vi "Practica1.vi"() -> ()   [LabVIEW 2021]
uses:
  <vilib>/imath/engines/lvmath2/RunTimeEngine/Managers/WorkSpace/UID Generator.vi
  <vilib>/imath/engines/lvmath2/RunTimeEngine/RunTimeType/NIMS_RunTimeType_From StrictType (excl LVString).vi
  <instcachedir>/0/NIMS_RunTimeType_From StrictType (excl LVString)_F2DF8362C4A748C4A5A87B97B2A722F9.lvgen/NIMS_RunTimeType_From StrictType (excl LVString)_F2DF8362C4A748C4A5A87B97B2A722F9_000.vi
  <vilib>/imath/engines/lvmath2/RunTimeEngine/LocalVariableDefStatement/MC_LocalVariableDefStatement_Display.vi
  <vilib>/imath/engines/lvmath2/RunTimeEngine/Managers/SymbolTable/Clear UID.vi
  <vilib>/imath/engines/lvmath2/RunTimeEngine/NodeEndStatement/NIMS_NodeEndStatement_Output.vi
  <instcachedir>/0/NIMS_NodeEndStatement_Output_53EC0D466D134D7ABD903AC30B43404B.lvgen/NIMS_NodeEndStatement_Output_53EC0D466D134D7ABD903AC30B43404B_001.vi
  <vilib>/imath/engines/lvmath2/RunTimeEngine/ErrorHandling/NIMS_Finalize Error.vi
  <vilib>/imath/engines/lvmath2/RunTimeEngine/ArithmeticOperatorToken/NIMS_ArithmeticOperator_power(S).vi
  <instcachedir>/0/NIMS_ArithmeticOperator_power(S)_149E20C93FA648E196B974450BC90546.lvgen/NIMS_ArithmeticOperator_power(S)_149E20C93FA648E196B974450BC90546_010.vi
  <vilib>/imathl/engines/lvmath/Functions/Error Handling/Create Error.vi
  <vilib>/imath/engines/lvmath2/RunTimeEngine/BuiltInFunctions/sin/NIMS_sin(C).vi
  <instcachedir>/0/NIMS_sin(C)_EF49EB6613814DD5AA1481177C690C0D.lvgen/NIMS_sin(C)_EF49EB6613814DD5AA1481177C690C0D_001.vi
  <vilib>/imath/engines/lvmath2/RunTimeEngine/BuiltInFunctions/cos/NIMS_cos(C).vi
  <instcachedir>/0/NIMS_cos(C)_035A4A914C7C4DF2869F8321D2939141.lvgen/NIMS_cos(C)_035A4A914C7C4DF2869F8321D2939141_001.vi
  <vilib>/imath/engines/lvmath2/RunTimeEngine/BuiltInFunctions/conv/NIMS_conv(V,V).vi
  <instcachedir>/0/NIMS_conv(V,V)_D3E194F2B5174935BB2368CEB7AAC5A9.lvgen/NIMS_conv(V,V)_D3E194F2B5174935BB2368CEB7AAC5A9_000.vi
  <vilib>/imath/engines/lvmath2/RunTimeEngine/ErrorHandling/NIMS_Error From Error Code.vi
  <vilib>/imath/engines/lvmath2/RunTimeEngine/IndexRead/NIMS V(S).vi
  <instcachedir>/0/NIMS V(S)_0488751826AF41519A22953C041130DC.lvgen/NIMS V(S)_0488751826AF41519A22953C041130DC_003.vi
  <vilib>/imath/engines/lvmath2/RunTimeEngine/ErrorHandling/NIMS_Create Error From Enums.vi
  <vilib>/imath/engines/lvmath2/RunTimeEngine/BuiltInFunctions/inv/NIMS_inv(GM).vi
  <instcachedir>/0/NIMS_inv(GM)_A6DF8FE880224208AACFE4CF9F659502.lvgen/NIMS_inv(GM)_A6DF8FE880224208AACFE4CF9F659502_001.vi
  <vilib>/imath/engines/lvmath2/RunTimeEngine/ArithmeticOperatorToken/NIMS_ArithmeticOperator_multmx(M,CV).vi
  <instcachedir>/0/NIMS_ArithmeticOperator_multmx(M,CV)_EA5705981BE742938BF830F3274AE397.lvgen/NIMS_ArithmeticOperator_multmx(M,CV)_EA5705981BE742938BF830F3274AE397_002.vi
  <vilib>/imath/engines/lvmath2/RunTimeEngine/IndexRead/NIMS M(S).vi
  <instcachedir>/0/NIMS M(S)_B826C018497E4940AE96BD27B540B6FB.lvgen/NIMS M(S)_B826C018497E4940AE96BD27B540B6FB_004.vi
  <instcachedir>/0/NIMS_NodeEndStatement_Output_53EC0D466D134D7ABD903AC30B43404B.lvgen/NIMS_NodeEndStatement_Output_53EC0D466D134D7ABD903AC30B43404B_009.vi
  <instcachedir>/0/NIMS_inv(GM)_A6DF8FE880224208AACFE4CF9F659502.lvgen/NIMS_inv(GM)_A6DF8FE880224208AACFE4CF9F659502_000.vi
  <instcachedir>/0/NIMS_ArithmeticOperator_multmx(M,CV)_EA5705981BE742938BF830F3274AE397.lvgen/NIMS_ArithmeticOperator_multmx(M,CV)_EA5705981BE742938BF830F3274AE397_000.vi
  <instcachedir>/0/NIMS M(S)_B826C018497E4940AE96BD27B540B6FB.lvgen/NIMS M(S)_B826C018497E4940AE96BD27B540B6FB_000.vi
  <vilib>/imath/engines/lvmath2/RunTimeEngine/Managers/SymbolTable/NIMS_WorkSpace.lvlib
panel:
  in  "Nivel \nPerturbación":dbl(slide) scale=0.0..100.0
  out "q2":dbl
  out "q1":dbl
  out "q0":dbl
  out "Salida LC":cdb
  out "Salida LA":dbl
  in  "Perturbación":bool
  out "Error":dbl
  in  "Selector":bool caption="Boolean"
  in  "a1":dbl=-0.678
  in  "b2":dbl=0.0168
  in  "b1":dbl=0.4592
  in  "Tm":dbl=0.04
  in  "Mp":dbl=10.0
  in  "tss":dbl=0.65
  in  "stop":bool
  in  "Set Point":dbl
  out "Sistema Controlado":T1(graph)
  # "Laboratorio Control Avanzado"
  # "Diseno de Controladores PI y PID por Asignación de Polos"
  # "Andrés Felipe Garavito González"
  # "Esteban Vásquez Cano"
  # "PID"
  # "z    +"
  # "HGp(z) = ----------------------------------"
  # "z^2   +"
  # "z"
  # "PI"
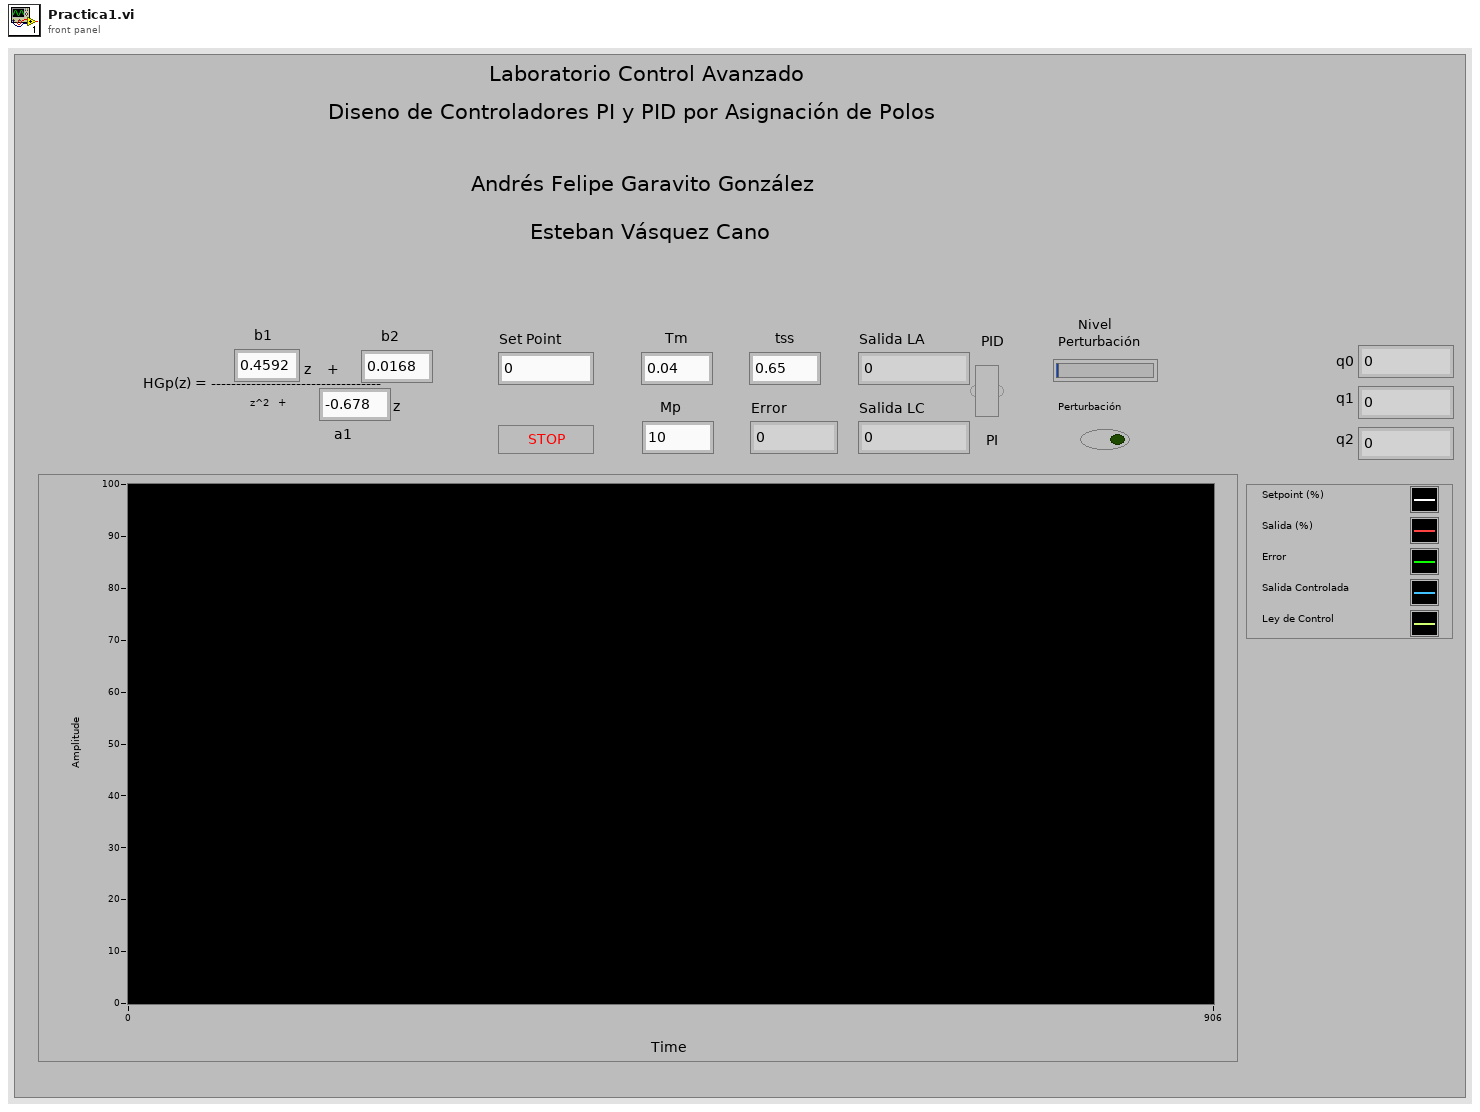
[diagram p1: front panel]
types:
  T1 = cluster{"Set Point U(k)":dbl, "yk":dbl, "Error":dbl, "ykc":dbl, "mk":dbl}
  T2 = cluster{"Set Point":dbl, "yk":dbl, cdb, cdb, "mk":cdb}
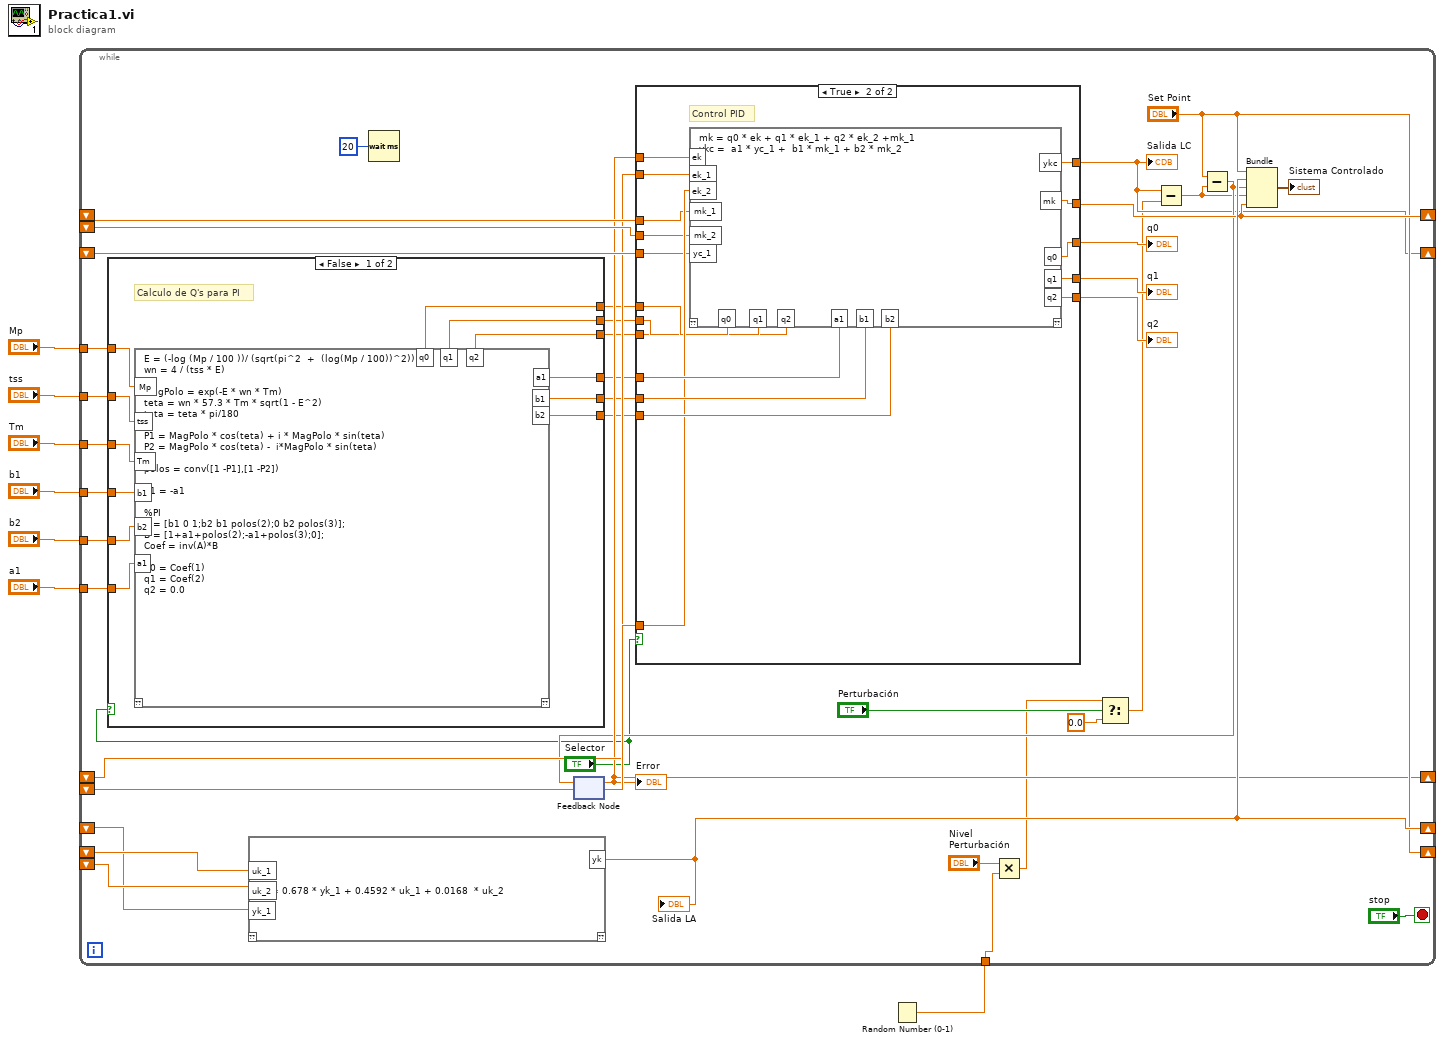
[diagram p0: block diagram]
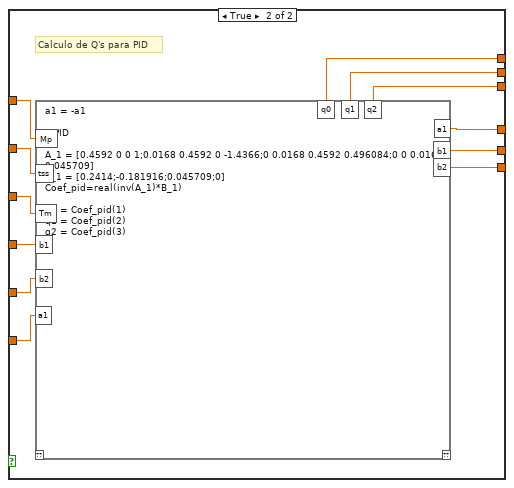
[diagram p2: hidden frame]
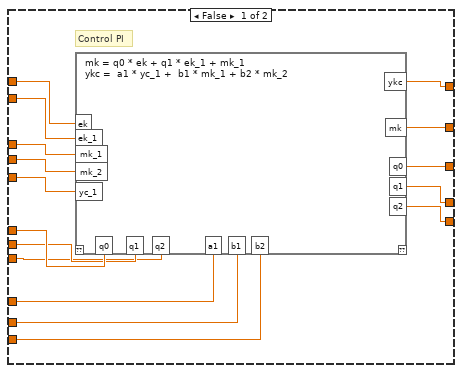
[diagram p3: hidden frame]
diagram:
  n1 = Random Number (0-1)() -> (number: 0 to 1=w1:dbl)
  n2 = while {
    shift-right: [w44] -> _
    shift-left: _ -> [w45]
    shift-right: ["Set Point"] -> _
    shift-left: _ -> [w47]
    shift-left: _ -> [w46]
    shift-right: [w37] -> _
    shift-left: _ -> [w41]
    shift-left: _ -> [w40]
    shift-right: [w27] -> _
    shift-left: _ -> [w39]
    shift-right: [w29] -> _
    shift-left: _ -> [w30]
    shift-left: _ -> [w36]
    tunnel: "Mp" -> [w24]
    tunnel: "tss" -> [w23]
    tunnel: "Tm" -> [w22]
    tunnel: "b1" -> [w21]
    tunnel: "b2" -> [w20]
    tunnel: "a1" -> [w19]
    tunnel: w1 -> [w10]
    stop <- "stop" stop-if-true
    n3 = case shown="False" "Selector" {
      tunnel: [w59 w503] -> w18
      tunnel: [w58 w502] -> w17
      tunnel: [w48 w501] -> w16
      tunnel: [w57 w500] -> w15
      tunnel: [w56 w499] -> w14
      tunnel: [w55 w498] -> w13
      tunnel: w24 -> [w54 w497]
      tunnel: w23 -> [w53 w496]
      tunnel: w22 -> [w52 w495]
      tunnel: w21 -> [w51 w494]
      tunnel: w20 -> [w50 w493]
      tunnel: w19 -> [w49 w492]
      frame False {
        # "Calculo de Q's para PI"
        n4 = mathscript code="E = (-log (Mp / 100 ))/ (sqrt(pi^2  +  (log(Mp / 100))^2))\nwn = 4 / (tss * E)\n\nMagPolo = exp(-E * wn * Tm)\nteta = wn * 57.3 * Tm * sqrt(1 - E^2)\nteta = teta * pi/180\n\nP1 = MagPolo * cos(teta) + i * MagPolo * sin(teta)\nP2 = MagPolo * cos(teta) -  i*MagPolo * sin(teta)\n\npolos = conv([1 -P1],[1 -P2])\n\na1 = -a1\n\n%PI\nA = [b1 0 1;b2 b1 polos(2);0 b2 polos(3)];\nB = [1+a1+polos(2);-a1+polos(3);0];\nCoef = inv(A)*B\n\nq0 = Coef(1)\nq1 = Coef(2)\nq2 = 0.0"("Mp"=w54, "tss"=w53, "Tm"=w52, "b1"=w51, "b2"=w50, "a1"=w49) -> ("q0"=w59:cdb, "q1"=w58:cdb, "a1"=w57:dbl, "b1"=w56:dbl, "b2"=w55:dbl, "q2"=w48:dbl)  [unwired: 1 in, 1 out]
      }
      frame True {
        # "Calculo de Q's para PID"
        n5 = mathscript code="a1 = -a1\n\n%PID\n\nA_1 = [0.4592 0 0 1;0.0168 0.4592 0 -1.4366;0 0.0168 0.4592 0.496084;0 0 0.0168 0.045709]\nB_1 = [0.2414;-0.181916;0.045709;0]\nCoef_pid=real(inv(A_1)*B_1)\n\nq0 = Coef_pid(1)\nq1 = Coef_pid(2)\nq2 = Coef_pid(3)"("Mp"=w497, "tss"=w496, "Tm"=w495, "b1"=w494, "b2"=w493, "a1"=w492) -> ("q0"=w503:dbl, "q1"=w502:dbl, "q2"=w501:dbl, "a1"=w500:dbl, "b1"=w499:dbl, "b2"=w498:dbl)  [unwired: 1 in, 1 out]
      }
    }
    n6 = mathscript code="yk = 0.678 * yk_1 + 0.4592 * uk_1 + 0.0168  * uk_2"("yk_1"=w45, "uk_1"=w47, "uk_2"=w46) -> ("yk"=w44:dbl)  [unwired: 1 in, 1 out]
    "Salida LA" <- w44
    n7 = Wait (ms)(milliseconds to wait=u32 20) -> ()  [unwired: 1 out]
    n8 = feedback #1() -> (w29:cdb)  [unwired: 1 in]
    "Error" <- w29
    n9 = case shown="True" "Selector" {
      tunnel: w29 -> [w713 w815]
      tunnel: w30 -> [w712 w816]
      tunnel: w41 -> [w711 w813]
      tunnel: w40 -> [w710 w812]
      tunnel: w39 -> [w709 w811]
      tunnel: [w707 w821] -> w27
      tunnel: [w708 w820] -> w37
      tunnel: w18 -> [w706 w807]
      tunnel: w17 -> [w705 w806]
      tunnel: w16 -> [w699 w805]
      tunnel: w15 -> [w704 w819]
      tunnel: w14 -> [w703 w818]
      tunnel: w13 -> [w702 w817]
      tunnel: w36 -> [_ w814]
      tunnel: [w701 w810] -> w34
      tunnel: [w700 w809] -> w33
      tunnel: [w698 w808] -> w32
      frame False {
        # "Control PI"
        n10 = mathscript code="mk = q0 * ek + q1 * ek_1 + mk_1\nykc =  a1 * yc_1 +  b1 * mk_1 + b2 * mk_2"("q1"=w705, "q0"=w706, "ek"=w713, "ek_1"=w712, "mk_1"=w711, "mk_2"=w710, "yc_1"=w709, "a1"=w704, "b1"=w703, "b2"=w702, "q2"=w699) -> ("mk"=w708:cdb, "ykc"=w707:cdb, "q0"=w701:cdb, "q1"=w700:cdb, "q2"=w698:dbl)  [unwired: 1 in, 1 out]
      }
      frame True {
        # "Control PID"
        n11 = mathscript code="mk = q0 * ek + q1 * ek_1 + q2 * ek_2 +mk_1\nykc =  a1 * yc_1 +  b1 * mk_1 + b2 * mk_2"("a1"=w819, "b1"=w818, "b2"=w817, "ek"=w815, "ek_1"=w816, "ek_2"=w814, "mk_1"=w813, "mk_2"=w812, "yc_1"=w811, "q0"=w807, "q1"=w806, "q2"=w805) -> ("mk"=w820:cdb, "ykc"=w821:cdb, "q0"=w810:cdb, "q1"=w809:cdb, "q2"=w808:dbl)  [unwired: 1 in, 1 out]
      }
    }
    "Salida LC" <- w27
    "q0" <- w34
    "q1" <- w33
    "q2" <- w32
    n12 = Multiply(x="Nivel \nPerturbación", y=w10) -> (x*y=w8:dbl)
    n13 = Select(t=w8, s="Perturbación", f=0.0) -> (s? t:f=w25:dbl)
    n14 = Subtract(x=w27, y=w25) -> (x-y=w26:cdb)
    n15 = Subtract(x="Set Point", y=w26) -> (x-y=w28:cdb)
    n16 = feedback-in #1(w28) -> ()
    n17 = Bundle("Set Point"="Set Point", "yk"=w44, w28, w26, "mk"=w37) -> (→"Sistema Controlado":T2)  [unwired: 1 in]
  }
